vi "Translator.vi"(0 "Input":variant, 11 "error in (no error)":errorcluster) -> (4 "Output":variant, 15 "error out":errorcluster)   [LabVIEW 2014, in "Arduino TFT.lvlib"]
doc: "An example of how to create the Translator to convert the LabVIEW VIs to Arduino C code."
uses:
  <vilib>/Aledyne-TSXperts/Arduino Compatible Compiler for LabVIEW/addons/Arduino TFT/Arduino TFT.lvlib
panel:
  out "Outputs":string[](array[string])
  out "Inputs":string[](array[string])
  out "Output Datatypes":string[](array[string])
  out "Input Datatypes":string[](array[string])
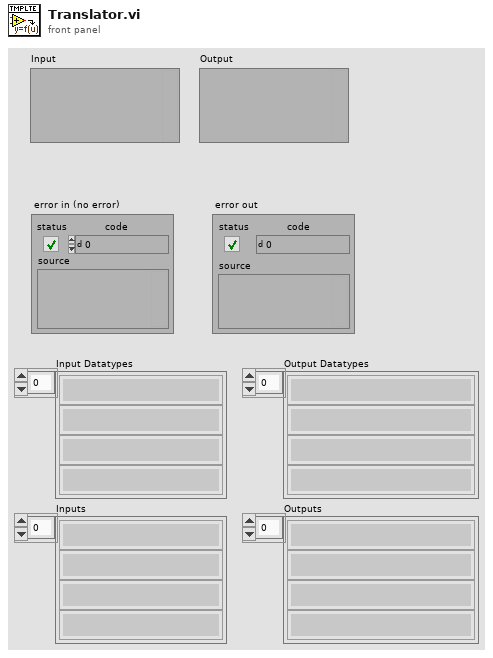
[diagram p1: front panel]
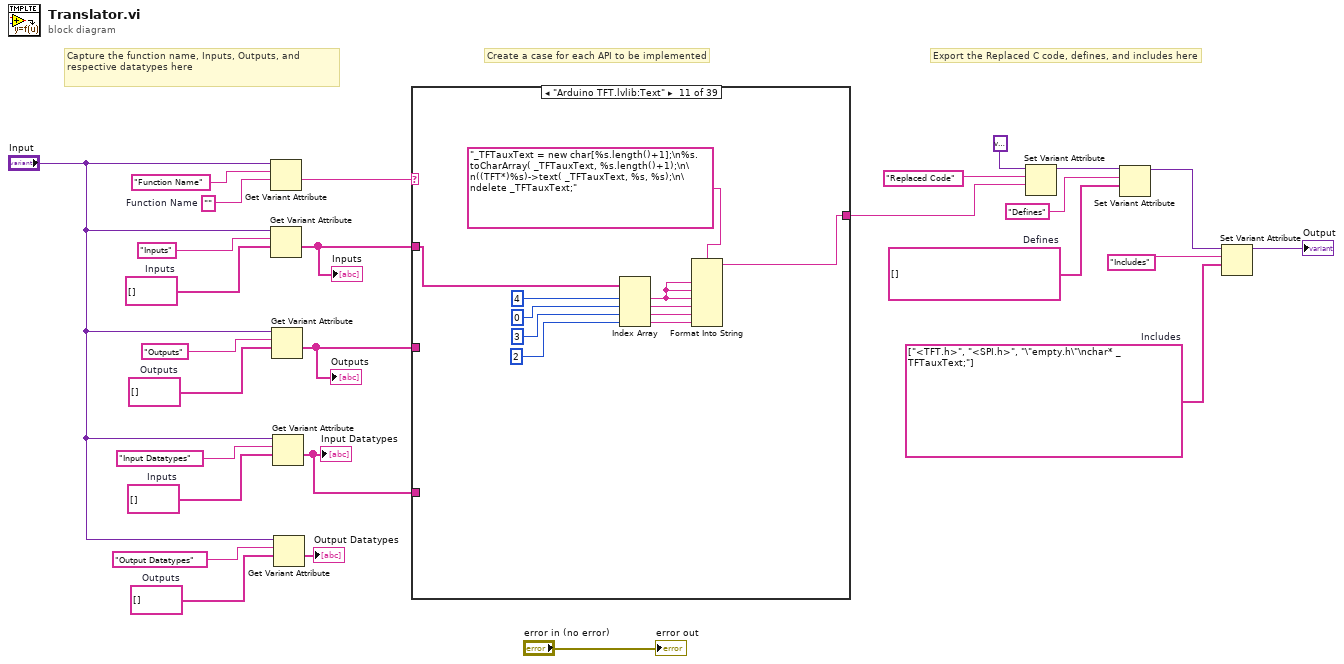
[diagram p0: block diagram]
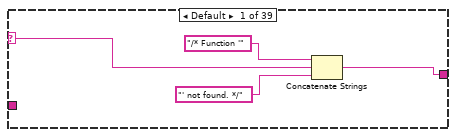
[diagram p2: hidden frame]
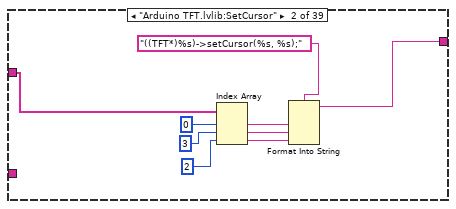
[diagram p3: hidden frame]
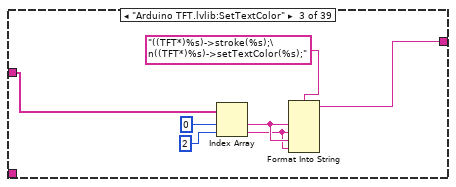
[diagram p4: hidden frame]
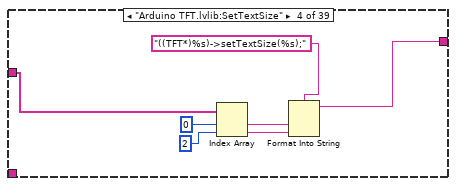
[diagram p5: hidden frame]
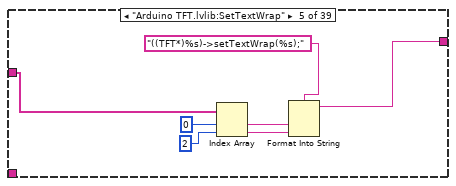
[diagram p6: hidden frame]
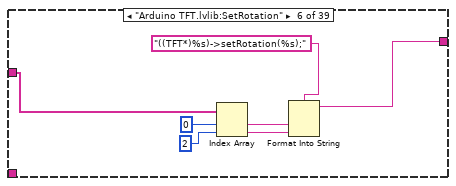
[diagram p7: hidden frame]
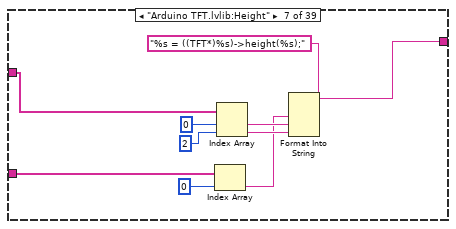
[diagram p8: hidden frame]
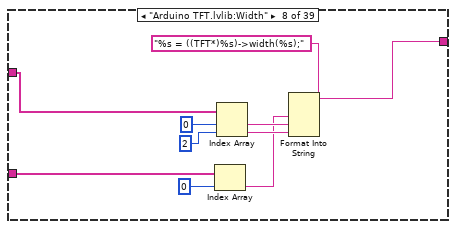
[diagram p9: hidden frame]
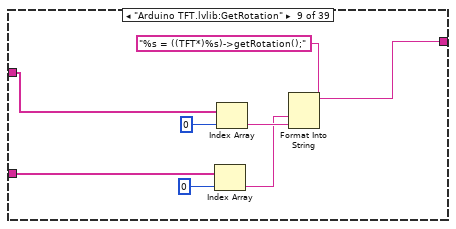
[diagram p10: hidden frame]
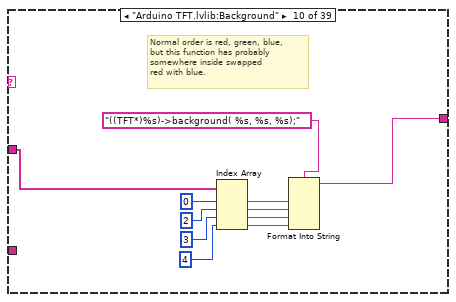
[diagram p11: hidden frame]
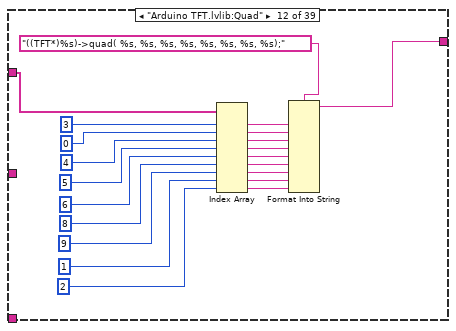
[diagram p12: hidden frame]
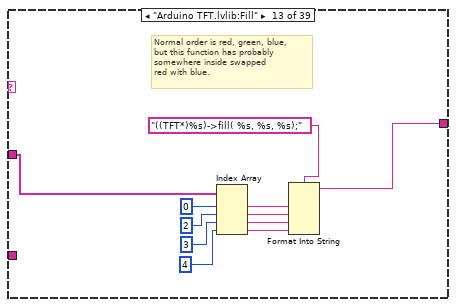
[diagram p13: hidden frame]
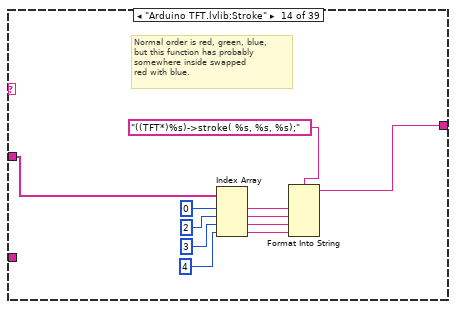
[diagram p14: hidden frame]
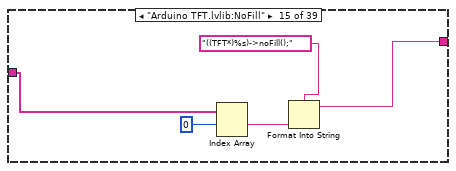
[diagram p15: hidden frame]
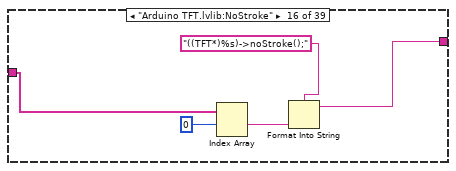
[diagram p16: hidden frame]
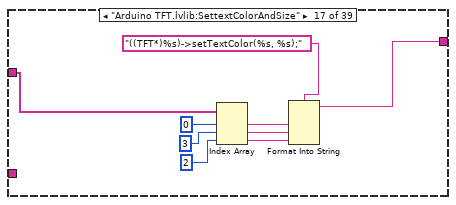
[diagram p17: hidden frame]
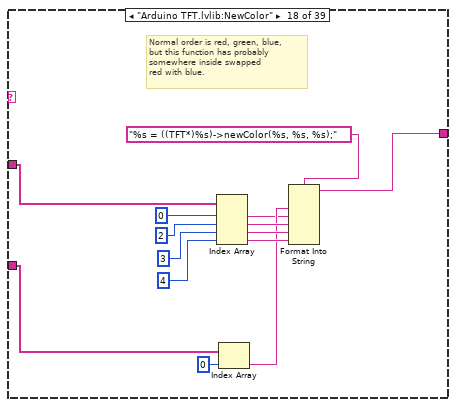
[diagram p18: hidden frame]
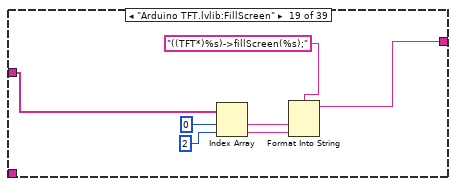
[diagram p19: hidden frame]
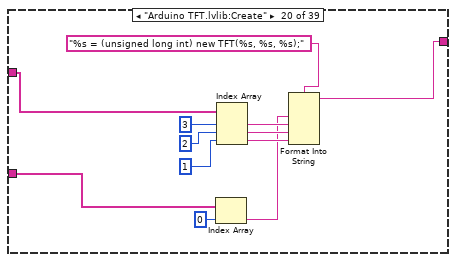
[diagram p20: hidden frame]
diagram:
  w2 = string[] []  # Defines
  w12 = string[] []  # Outputs
  w13 = string[] []  # Inputs
  w18 = string[] ["<TFT.h>", "<SPI.h>", "\"empty.h\"\nchar* _TFTauxText;"]  # Includes
  w23 = string[] []  # Outputs
  w24 = string[] []  # Inputs
  w25 = ""  # Function Name
  # "Capture the function name, Inputs, Outputs, and respective datatypes here"
  # "Export the Replaced C code, defines, and includes here"
  # "Create a case for each API to be implemented"
  n1 = Get Variant Attribute(Variant="Input", name="Function Name", default value (empty Variant)=w25) -> (value=w20:string)  [unwired: 1 in, 3 out]
  n2 = Get Variant Attribute(Variant="Input", name="Inputs", default value (empty Variant)=w24) -> (value=w7:string[])  [unwired: 1 in, 3 out]
  "Inputs" <- w7
  n3 = Get Variant Attribute(Variant="Input", name="Outputs", default value (empty Variant)=w23) -> (value=w8:string[])  [unwired: 1 in, 3 out]
  "Outputs" <- w8
  n4 = Get Variant Attribute(Variant="Input", name="Input Datatypes", default value (empty Variant)=w13) -> (value=w1:string[])  [unwired: 1 in, 3 out]
  "Input Datatypes" <- w1
  n5 = Get Variant Attribute(Variant="Input", name="Output Datatypes", default value (empty Variant)=w12) -> (value=→"Output Datatypes":string[])  [unwired: 1 in, 3 out]
  n6 = case shown="\"Arduino TFT.lvlib:Text\"" w20 {
    selector: w20 -> [w30 _ _ _ _ _ _ _ _ _ _ _ _ _ _ _ _ _ _ _ _ _ _ _ _ _ _ _ _ _ _ _ _ _ _ _ _ _ _]
    tunnel: [w28 w36 w43 w50 w57 w64 w74 w84 w93 w104 w115 w136 w147 w158 w163 w168 w176 w191 w197 w209 w220 w229 w242 w255 w268 w279 w292 w307 w320 w335 w348 w365 w382 w401 w420 w435 w452 w469 w475] -> w19
    tunnel: w7 -> [_ w40 w47 w54 w61 w68 w78 w88 w96 w107 w118 w139 w150 w161 w166 w171 w180 w194 w201 w213 w224 w233 w246 w259 w272 w283 w296 w311 w324 w339 w352 w369 w386 w405 w424 w439 w456 w473 w478]
    tunnel: w8 -> [_ _ _ _ _ _ w69 w79 w89 _ _ _ _ _ _ _ _ w186 _ w204 _ _ _ _ _ _ _ _ _ _ _ _ _ _ _ _ _ _ _]
    tunnel: w1 -> [_ _ _ _ _ _ _ _ _ _ _ _ _ _ _ _ _ _ _ _ _ _ _ _ _ _ _ _ _ _ _ _ _ _ _ _ _ _ _]
    frame Default {
      n7 = Concatenate Strings("/* Function '", w30, "' not found. */") -> (w28:string)
    }
    frame "Arduino TFT.lvlib:SetCursor" {
      n8 = Index Array(array=w40, index #1=0 ("index"), index #2=3 ("index"), index #3=2 ("index")) -> (element #1=w34:string, element #2=w33:string, element #3=w32:string)
      n9 = Format Into String(format string="((TFT*)%s)->setCursor(%s, %s);", w34, w33, w32) -> (resulting string=w36:string)  [unwired: 2 in, 1 out]
    }
    frame "Arduino TFT.lvlib:SetTextColor" {
      n10 = Index Array(array=w47, index #1=0 ("index"), index #2=2 ("index")) -> (element #1=w42:string, element #2=w41:string)
      n11 = Format Into String(format string="((TFT*)%s)->stroke(%s);\n((TFT*)%s)->setTextColor(%s);", w42, w41, w42, w41) -> (resulting string=w43:string)  [unwired: 2 in, 1 out]
    }
    frame "Arduino TFT.lvlib:SetTextSize" {
      n12 = Index Array(array=w54, index #1=0 ("index"), index #2=2 ("index")) -> (element #1=w49:string, element #2=w48:string)
      n13 = Format Into String(format string="((TFT*)%s)->setTextSize(%s);", w49, w48) -> (resulting string=w50:string)  [unwired: 2 in, 1 out]
    }
    frame "Arduino TFT.lvlib:SetTextWrap" {
      n14 = Index Array(array=w61, index #1=0 ("index"), index #2=2 ("index")) -> (element #1=w56:string, element #2=w55:string)
      n15 = Format Into String(format string="((TFT*)%s)->setTextWrap(%s);", w56, w55) -> (resulting string=w57:string)  [unwired: 2 in, 1 out]
    }
    frame "Arduino TFT.lvlib:SetRotation" {
      n16 = Index Array(array=w68, index #1=0 ("index"), index #2=2 ("index")) -> (element #1=w63:string, element #2=w62:string)
      n17 = Format Into String(format string="((TFT*)%s)->setRotation(%s);", w63, w62) -> (resulting string=w64:string)  [unwired: 2 in, 1 out]
    }
    frame "Arduino TFT.lvlib:Height" {
      n18 = Index Array(array=w69, index=0) -> (element=w70:string)
      n19 = Index Array(array=w78, index #1=0 ("index"), index #2=2 ("index")) -> (element #1=w73:string, element #2=w72:string)
      n20 = Format Into String(format string="%s = ((TFT*)%s)->height(%s);", w70, w73, w72) -> (resulting string=w74:string)  [unwired: 2 in, 1 out]
    }
    frame "Arduino TFT.lvlib:Width" {
      n21 = Index Array(array=w79, index=0) -> (element=w80:string)
      n22 = Index Array(array=w88, index #1=0 ("index"), index #2=2 ("index")) -> (element #1=w83:string, element #2=w82:string)
      n23 = Format Into String(format string="%s = ((TFT*)%s)->width(%s);", w80, w83, w82) -> (resulting string=w84:string)  [unwired: 2 in, 1 out]
    }
    frame "Arduino TFT.lvlib:GetRotation" {
      n24 = Index Array(array=w89, index=0) -> (element=w90:string)
      n25 = Index Array(array=w96, index=0) -> (element=w92:string)
      n26 = Format Into String(format string="%s = ((TFT*)%s)->getRotation();", w90, w92) -> (resulting string=w93:string)  [unwired: 2 in, 1 out]
    }
    frame "Arduino TFT.lvlib:Background" {
      # "Normal order is red, green, blue,\nbut this function has probably\nsomewhere inside swapped\nred with blue."
      n27 = Index Array(array=w107, index #1=0 ("index"), index #2=2 ("index"), index #3=3 ("index"), index #4=4 ("index")) -> (element #1=w103:string, element #2=w99:string, element #3=w98:string, element #4=w97:string)
      n28 = Format Into String(format string="((TFT*)%s)->background( %s, %s, %s);", w103, w99, w98, w97) -> (resulting string=w104:string)  [unwired: 2 in, 1 out]
    }
    frame "Arduino TFT.lvlib:Text" {
      n29 = Index Array(array=w118, index #1=4 ("index"), index #2=0 ("index"), index #3=3 ("index"), index #4=2 ("index")) -> (element #1=w108:string, element #2=w109:string, element #3=w111:string, element #4=w110:string)
      n30 = Format Into String(format string="_TFTauxText = new char[%s.length()+1];\n%s.toCharArray( _TFTauxText, %s.length()+1);\n\n((TFT*)%s)->text( _TFTauxText, %s, %s);\n\ndelete _TFTauxText;", w108, w108, w108, w109, w111, w110) -> (resulting string=w115:string)  [unwired: 2 in, 1 out]
    }
    frame "Arduino TFT.lvlib:Quad" {
      n31 = Index Array(array=w139, index #1=3 ("index"), index #2=0 ("index"), index #3=4 ("index"), index #4=5 ("index"), index #5=6 ("index"), index #6=8 ("index"), index #7=9 ("index"), index #8=1 ("index"), index #9=2 ("index")) -> (element #1=w135:string, element #2=w134:string, element #3=w133:string, element #4=w132:string, element #5=w123:string, element #6=w122:string, element #7=w121:string, element #8=w120:string, element #9=w119:string)
      n32 = Format Into String(format string="((TFT*)%s)->quad( %s, %s, %s, %s, %s, %s, %s, %s);", w135, w134, w133, w132, w123, w122, w121, w120, w119) -> (resulting string=w136:string)  [unwired: 2 in, 1 out]
    }
    frame "Arduino TFT.lvlib:Fill" {
      # "Normal order is red, green, blue,\nbut this function has probably\nsomewhere inside swapped\nred with blue."
      n33 = Index Array(array=w150, index #1=0 ("index"), index #2=2 ("index"), index #3=3 ("index"), index #4=4 ("index")) -> (element #1=w146:string, element #2=w142:string, element #3=w141:string, element #4=w140:string)
      n34 = Format Into String(format string="((TFT*)%s)->fill( %s, %s, %s);", w146, w142, w141, w140) -> (resulting string=w147:string)  [unwired: 2 in, 1 out]
    }
    frame "Arduino TFT.lvlib:Stroke" {
      # "Normal order is red, green, blue,\nbut this function has probably\nsomewhere inside swapped\nred with blue."
      n35 = Index Array(array=w161, index #1=0 ("index"), index #2=2 ("index"), index #3=3 ("index"), index #4=4 ("index")) -> (element #1=w157:string, element #2=w153:string, element #3=w152:string, element #4=w151:string)
      n36 = Format Into String(format string="((TFT*)%s)->stroke( %s, %s, %s);", w157, w153, w152, w151) -> (resulting string=w158:string)  [unwired: 2 in, 1 out]
    }
    frame "Arduino TFT.lvlib:NoFill" {
      n37 = Index Array(array=w166, index #1=0 ("index")) -> (element #1=w162:string)  [unwired: 1 in, 1 out]
      n38 = Format Into String(format string="((TFT*)%s)->noFill();", w162) -> (resulting string=w163:string)  [unwired: 2 in, 1 out]
    }
    frame "Arduino TFT.lvlib:NoStroke" {
      n39 = Index Array(array=w171, index #1=0 ("index")) -> (element #1=w167:string)  [unwired: 1 in, 1 out]
      n40 = Format Into String(format string="((TFT*)%s)->noStroke();", w167) -> (resulting string=w168:string)  [unwired: 2 in, 1 out]
    }
    frame "Arduino TFT.lvlib:SettextColorAndSize" {
      n41 = Index Array(array=w180, index #1=0 ("index"), index #2=3 ("index"), index #3=2 ("index")) -> (element #1=w175:string, element #2=w174:string, element #3=w173:string)
      n42 = Format Into String(format string="((TFT*)%s)->setTextColor(%s, %s);", w175, w174, w173) -> (resulting string=w176:string)  [unwired: 2 in, 1 out]
    }
    frame "Arduino TFT.lvlib:NewColor" {
      # "Normal order is red, green, blue,\nbut this function has probably\nsomewhere inside swapped\nred with blue."
      n43 = Index Array(array=w194, index #1=0 ("index"), index #2=2 ("index"), index #3=3 ("index"), index #4=4 ("index")) -> (element #1=w181:string, element #2=w189:string, element #3=w188:string, element #4=w184:string)
      n44 = Index Array(array=w186, index=0) -> (element=w182:string)
      n45 = Format Into String(format string="%s = ((TFT*)%s)->newColor(%s, %s, %s);", w182, w181, w189, w188, w184) -> (resulting string=w191:string)  [unwired: 2 in, 1 out]
    }
    frame "Arduino TFT.lvlib:FillScreen" {
      n46 = Index Array(array=w201, index #1=0 ("index"), index #2=2 ("index")) -> (element #1=w196:string, element #2=w195:string)
      n47 = Format Into String(format string="((TFT*)%s)->fillScreen(%s);", w196, w195) -> (resulting string=w197:string)  [unwired: 2 in, 1 out]
    }
    frame "Arduino TFT.lvlib:Create" {
      n48 = Index Array(array=w204, index=0) -> (element=w203:string)
      n49 = Index Array(array=w213, index #1=3 ("index"), index #2=2 ("index"), index #3=1 ("index")) -> (element #1=w207:string, element #2=w206:string, element #3=w205:string)
      n50 = Format Into String(format string="%s = (unsigned long int) new TFT(%s, %s, %s);", w203, w207, w206, w205) -> (resulting string=w209:string)  [unwired: 2 in, 1 out]
    }
    frame "Arduino TFT.lvlib:DrawPixel" {
      n51 = Index Array(array=w224, index #1=0 ("index"), index #2=4 ("index"), index #3=3 ("index"), index #4=2 ("index")) -> (element #1=w218:string, element #2=w217:string, element #3=w216:string, element #4=w214:string)
      n52 = Format Into String(format string="((TFT*)%s)->drawPixel(%s, %s, %s);", w218, w217, w216, w214) -> (resulting string=w220:string)  [unwired: 2 in, 1 out]
    }
    frame "Arduino TFT.lvlib:Point" {
      n53 = Index Array(array=w233, index #1=0 ("index"), index #2=3 ("index"), index #3=2 ("index")) -> (element #1=w227:string, element #2=w226:string, element #3=w225:string)
      n54 = Format Into String(format string="((TFT*)%s)->point(%s, %s);", w227, w226, w225) -> (resulting string=w229:string)  [unwired: 2 in, 1 out]
    }
    frame "Arduino TFT.lvlib:DrawFastVLine" {
      n55 = Index Array(array=w246, index #1=0 ("index"), index #2=5 ("index"), index #3=4 ("index"), index #4=3 ("index"), index #5=1 ("index")) -> (element #1=w240:string, element #2=w239:string, element #3=w238:string, element #4=w236:string, element #5=w234:string)
      n56 = Format Into String(format string="((TFT*)%s)->drawFastVLine(%s, %s, %s, %s);", w240, w239, w238, w236, w234) -> (resulting string=w242:string)  [unwired: 2 in, 1 out]
    }
    frame "Arduino TFT.lvlib:DrawFastHLine" {
      n57 = Index Array(array=w259, index #1=0 ("index"), index #2=5 ("index"), index #3=4 ("index"), index #4=3 ("index"), index #5=1 ("index")) -> (element #1=w253:string, element #2=w252:string, element #3=w251:string, element #4=w249:string, element #5=w247:string)
      n58 = Format Into String(format string="((TFT*)%s)->drawFastHLine(%s, %s, %s, %s);", w253, w252, w251, w249, w247) -> (resulting string=w255:string)  [unwired: 2 in, 1 out]
    }
    frame "Arduino TFT.lvlib:DrawCircle" {
      n59 = Index Array(array=w272, index #1=0 ("index"), index #2=5 ("index"), index #3=4 ("index"), index #4=3 ("index"), index #5=1 ("index")) -> (element #1=w266:string, element #2=w265:string, element #3=w264:string, element #4=w262:string, element #5=w260:string)
      n60 = Format Into String(format string="((TFT*)%s)->drawCircle(%s, %s, %s, %s);", w266, w265, w264, w262, w260) -> (resulting string=w268:string)  [unwired: 2 in, 1 out]
    }
    frame "Arduino TFT.lvlib:Circle" {
      n61 = Index Array(array=w283, index #1=0 ("index"), index #2=4 ("index"), index #3=3 ("index"), index #4=2 ("index")) -> (element #1=w277:string, element #2=w276:string, element #3=w275:string, element #4=w273:string)
      n62 = Format Into String(format string="((TFT*)%s)->circle(%s, %s, %s);", w277, w276, w275, w273) -> (resulting string=w279:string)  [unwired: 2 in, 1 out]
    }
    frame "Arduino TFT.lvlib:FillCircle" {
      n63 = Index Array(array=w296, index #1=0 ("index"), index #2=5 ("index"), index #3=4 ("index"), index #4=3 ("index"), index #5=1 ("index")) -> (element #1=w290:string, element #2=w289:string, element #3=w288:string, element #4=w286:string, element #5=w284:string)
      n64 = Format Into String(format string="((TFT*)%s)->fillCircle(%s, %s, %s, %s);", w290, w289, w288, w286, w284) -> (resulting string=w292:string)  [unwired: 2 in, 1 out]
    }
    frame "Arduino TFT.lvlib:DrawLine" {
      n65 = Index Array(array=w311, index #1=2 ("index"), index #2=0 ("index"), index #3=3 ("index"), index #4=4 ("index"), index #5=5 ("index"), index #6=1 ("index")) -> (element #1=w297:string, element #2=w305:string, element #3=w304:string, element #4=w303:string, element #5=w301:string, element #6=w299:string)
      n66 = Format Into String(format string="((TFT*)%s)->drawLine(%s, %s, %s, %s, %s);", w297, w305, w304, w303, w301, w299) -> (resulting string=w307:string)  [unwired: 2 in, 1 out]
    }
    frame "Arduino TFT.lvlib:Line" {
      n67 = Index Array(array=w324, index #1=1 ("index"), index #2=0 ("index"), index #3=2 ("index"), index #4=3 ("index"), index #5=4 ("index")) -> (element #1=w312:string, element #2=w318:string, element #3=w317:string, element #4=w316:string, element #5=w314:string)
      n68 = Format Into String(format string="((TFT*)%s)->line(%s, %s, %s, %s);", w312, w318, w317, w316, w314) -> (resulting string=w320:string)  [unwired: 2 in, 1 out]
    }
    frame "Arduino TFT.lvlib:DrawRect" {
      n69 = Index Array(array=w339, index #1=2 ("index"), index #2=0 ("index"), index #3=3 ("index"), index #4=4 ("index"), index #5=5 ("index"), index #6=1 ("index")) -> (element #1=w325:string, element #2=w333:string, element #3=w332:string, element #4=w331:string, element #5=w329:string, element #6=w327:string)
      n70 = Format Into String(format string="((TFT*)%s)->drawRect(%s, %s, %s, %s, %s);", w325, w333, w332, w331, w329, w327) -> (resulting string=w335:string)  [unwired: 2 in, 1 out]
    }
    frame "Arduino TFT.lvlib:Rect" {
      n71 = Index Array(array=w352, index #1=1 ("index"), index #2=0 ("index"), index #3=2 ("index"), index #4=3 ("index"), index #5=4 ("index")) -> (element #1=w340:string, element #2=w346:string, element #3=w345:string, element #4=w344:string, element #5=w342:string)
      n72 = Format Into String(format string="((TFT*)%s)->rect(%s, %s, %s, %s);", w340, w346, w345, w344, w342) -> (resulting string=w348:string)  [unwired: 2 in, 1 out]
    }
    frame "Arduino TFT.lvlib:DrawBitmap" {
      n73 = Index Array(array=w369, index #1=3 ("index"), index #2=0 ("index"), index #3=4 ("index"), index #4=2 ("index"), index #5=5 ("index"), index #6=6 ("index"), index #7=1 ("index")) -> (element #1=w355:string, element #2=w363:string, element #3=w362:string, element #4=w361:string, element #5=w359:string, element #6=w357:string, element #7=w353:string)
      n74 = Format Into String(format string="((TFT*)%s)->drawBitmap(%s, %s, %s, %s, %s, %s);", w355, w363, w362, w361, w359, w357, w353) -> (resulting string=w365:string)  [unwired: 2 in, 1 out]
    }
    frame "Arduino TFT.lvlib:DrawChar" {
      n75 = Index Array(array=w386, index #1=3 ("index"), index #2=0 ("index"), index #3=4 ("index"), index #4=1 ("index"), index #5=2 ("index"), index #6=9 ("index"), index #7=8 ("index")) -> (element #1=w372:string, element #2=w380:string, element #3=w379:string, element #4=w378:string, element #5=w376:string, element #6=w374:string, element #7=w370:string)
      n76 = Format Into String(format string="((TFT*)%s)->drawChar(%s, %s, %s, %s, %s, %s);", w372, w380, w379, w378, w376, w374, w370) -> (resulting string=w382:string)  [unwired: 2 in, 1 out]
    }
    frame "Arduino TFT.lvlib:DrawTriangle" {
      n77 = Index Array(array=w405, index #1=2 ("index"), index #2=0 ("index"), index #3=3 ("index"), index #4=4 ("index"), index #5=5 ("index"), index #6=7 ("index"), index #7=8 ("index"), index #8=1 ("index")) -> (element #1=w391:string, element #2=w399:string, element #3=w398:string, element #4=w397:string, element #5=w395:string, element #6=w393:string, element #7=w388:string, element #8=w387:string)
      n78 = Format Into String(format string="((TFT*)%s)->drawTriangle(%s, %s, %s, %s, %s, %s, %s);", w391, w399, w398, w397, w395, w393, w388, w387) -> (resulting string=w401:string)  [unwired: 2 in, 1 out]
    }
    frame "Arduino TFT.lvlib:FillTriangle" {
      n79 = Index Array(array=w424, index #1=2 ("index"), index #2=0 ("index"), index #3=3 ("index"), index #4=4 ("index"), index #5=5 ("index"), index #6=7 ("index"), index #7=8 ("index"), index #8=1 ("index")) -> (element #1=w410:string, element #2=w418:string, element #3=w417:string, element #4=w416:string, element #5=w414:string, element #6=w412:string, element #7=w407:string, element #8=w406:string)
      n80 = Format Into String(format string="((TFT*)%s)->fillTriangle(%s, %s, %s, %s, %s, %s, %s);", w410, w418, w417, w416, w414, w412, w407, w406) -> (resulting string=w420:string)  [unwired: 2 in, 1 out]
    }
    frame "Arduino TFT.lvlib:FillRect" {
      n81 = Index Array(array=w439, index #1=2 ("index"), index #2=0 ("index"), index #3=3 ("index"), index #4=4 ("index"), index #5=5 ("index"), index #6=1 ("index")) -> (element #1=w425:string, element #2=w433:string, element #3=w432:string, element #4=w431:string, element #5=w429:string, element #6=w427:string)
      n82 = Format Into String(format string="((TFT*)%s)->fillRect(%s, %s, %s, %s, %s);", w425, w433, w432, w431, w429, w427) -> (resulting string=w435:string)  [unwired: 2 in, 1 out]
    }
    frame "Arduino TFT.lvlib:DrawRoundRect" {
      n83 = Index Array(array=w456, index #1=3 ("index"), index #2=0 ("index"), index #3=4 ("index"), index #4=5 ("index"), index #5=6 ("index"), index #6=1 ("index"), index #7=2 ("index")) -> (element #1=w442:string, element #2=w450:string, element #3=w449:string, element #4=w448:string, element #5=w446:string, element #6=w444:string, element #7=w440:string)
      n84 = Format Into String(format string="((TFT*)%s)->drawRoundRect(%s, %s, %s, %s, %s, %s);", w442, w450, w449, w448, w446, w444, w440) -> (resulting string=w452:string)  [unwired: 2 in, 1 out]
    }
    frame "Arduino TFT.lvlib:FillRoundRect" {
      n85 = Index Array(array=w473, index #1=3 ("index"), index #2=0 ("index"), index #3=4 ("index"), index #4=5 ("index"), index #5=6 ("index"), index #6=1 ("index"), index #7=2 ("index")) -> (element #1=w459:string, element #2=w467:string, element #3=w466:string, element #4=w465:string, element #5=w463:string, element #6=w461:string, element #7=w457:string)
      n86 = Format Into String(format string="((TFT*)%s)->fillRoundRect(%s, %s, %s, %s, %s, %s);", w459, w467, w466, w465, w463, w461, w457) -> (resulting string=w469:string)  [unwired: 2 in, 1 out]
    }
    frame "Arduino TFT.lvlib:Begin" {
      n87 = Index Array(array=w478, index=1) -> (element=w474:string)
      n88 = Format Into String(format string="((TFT*)%s)->begin();", w474) -> (resulting string=w475:string)  [unwired: 2 in, 1 out]
    }
  }
  n89 = Set Variant Attribute(Variant=variant ("variant"), name="Replaced Code", value=w19) -> (Variant out=w5:variant)  [unwired: 1 in, 2 out]
  n90 = Set Variant Attribute(Variant=w5, name="Defines", value=w2) -> (Variant out=w4:variant)  [unwired: 1 in, 2 out]
  n91 = Set Variant Attribute(Variant=w4, name="Includes", value=w18) -> (Variant out=→"Output":variant)  [unwired: 1 in, 2 out]
  "error out" <- "error in (no error)"
